vi "Constructor.vi"(11 "Visible":bool) -> (3 "Excel Interface out":refnum<class "Excel Interface.lvclass">)   [LabVIEW 2016, in "Excel Interface.lvclass"]
uses:
  Excel Interface.lvclass
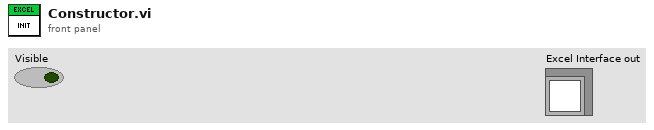
[diagram p1: front panel]
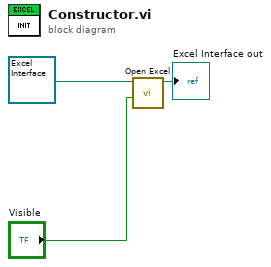
[diagram p0: block diagram]
diagram:
  n1 = call-dynamic "Open Excel.vi"("Visible"="Visible", "Excel Interface in"=refnum<class "Excel Interface.lvclass"> refnum ("Excel Interface.lvclass")) -> ("Excel Interface out"=→"Excel Interface out":refnum<class "Excel Interface.lvclass">)  [unwired: 8 in, 1 out]
